vi "Test.vi"() -> ()   [LabVIEW 2009]
panel:
  out "dequeued element":string
  out "x = y?":bool
  out "element":string
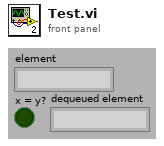
[diagram p1: front panel]
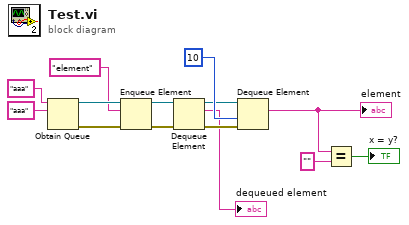
[diagram p0: block diagram]
diagram:
  n1 = Obtain Queue(name (unnamed)="aaa", element data type="aaa" ("name (unnamed)")) -> (queue out=w12:refnum<queue>, error out=w6:errorcluster)  [unwired: 3 in, 1 out]
  n2 = Enqueue Element(queue=w12, element="element", error in (no error)=w6) -> (queue out=w7:refnum<queue>, error out=w3:errorcluster)  [unwired: 1 in, 1 out]
  n3 = Dequeue Element(queue=w7, error in (no error)=w3) -> (queue out=w4:refnum<queue>, element=→"dequeued element":string, error out=w2:errorcluster)  [unwired: 1 in, 1 out]
  n4 = Dequeue Element(queue=w4, timeout in ms (-1)=10, error in (no error)=w2) -> (element=w10:string)  [unwired: 3 out]
  "element" <- w10
  n5 = Equal?(x=w10, y="") -> (x = y?=→"x = y?":bool)
